vi "Naplók_mappa.vi"() -> (3 "*\\Naplók útvonala":path)   [LabVIEW 2014]
doc: "Az *\\Naplók mappa útvonalának összeállítása."
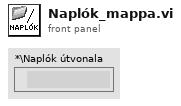
[diagram p1: front panel]
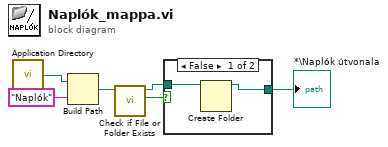
[diagram p0: block diagram]
diagram:
  n1 = call <vilib>:"Application Directory.vi"() -> ("Application Directory"=w6:path)
  n2 = Build Path(base path=w6, name or relative path="Naplók") -> (appended path=w4:path)
  n3 = call <vilib>:"Check if File or Folder Exists.vi"("path"=w4) -> ("file or folder exists?"=w3:bool, "dup path"=w2:path)  [unwired: 8 in, 1 out]
  n4 = case shown="False" w3 {
    tunnel: w2 -> [w8 w9]
    tunnel: [w7 w9] -> w1
    frame False {
      n5 = Create Folder(path (use dialog)=w8) -> (created path=w7:path)  [unwired: 2 in, 2 out]
    }
    frame True {
    }
  }
  "*\\Naplók útvonala" <- w1
